vi "Build Signal name.vi"(9 "Added Name":string, 10 "Units":string, 11 "Signal Name":string) -> (3 "Output":string[](array[string]))   [LabVIEW 2019]
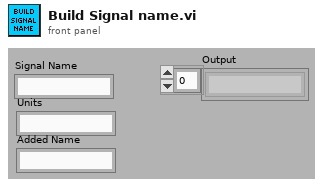
[diagram p1: front panel]
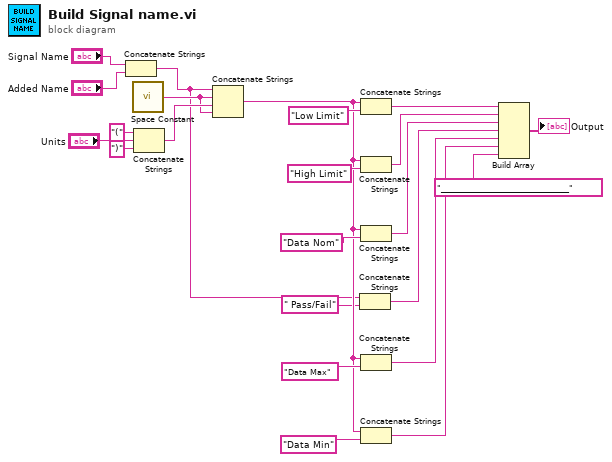
[diagram p0: block diagram]
diagram:
  n1 = Concatenate Strings("Signal Name", "Added Name") -> (w1:string)
  n2 = call <vilib>:"Space Constant.vi"() -> ("String"=w5:string)
  n3 = Concatenate Strings("(" ("string"), "Units", ")" ("string")) -> (w13:string)
  n4 = Concatenate Strings(w1, w5, w13, w5) -> (w4:string)
  n5 = Concatenate Strings(w1, " Pass/Fail") -> (w2:string)
  n6 = Concatenate Strings(w4, "Low Limit") -> (w12:string)
  n7 = Concatenate Strings(w4, "High Limit") -> (w11:string)
  n8 = Concatenate Strings(w4, "Data Nom") -> (w10:string)
  n9 = Concatenate Strings(w4, "Data Max") -> (w9:string)
  n10 = Concatenate Strings(w4, "Data Min") -> (w8:string)
  n11 = Build Array(w12, w11, w10, w2, w9, w8, "________________________________" ("element")) -> (→"Output":string[])
